vi "INI_Driver.vi"(0 "Data_In":string, 1 "Config_File_Path":path, 2 "Section":string, 5 "Key":string, 11 "Error_Out":errorcluster, 13 "INI_Operation_Select":T1=enum."Write") -> (4 "Data_Out":string, 6 "Key_Names":string[](array[string]), 15 "Error_Out":errorcluster)   [LabVIEW 2023]
doc: "Used to read and write the ini file"
uses:
  Controls/INI_Operation_Select.ctl
  <vilib>/Utility/config.llb/Read Key (String).vi
  <vilib>/Utility/config.llb/Write Key (String).vi
  <vilib>/Utility/config.llb/NI_LVConfig.lvlib
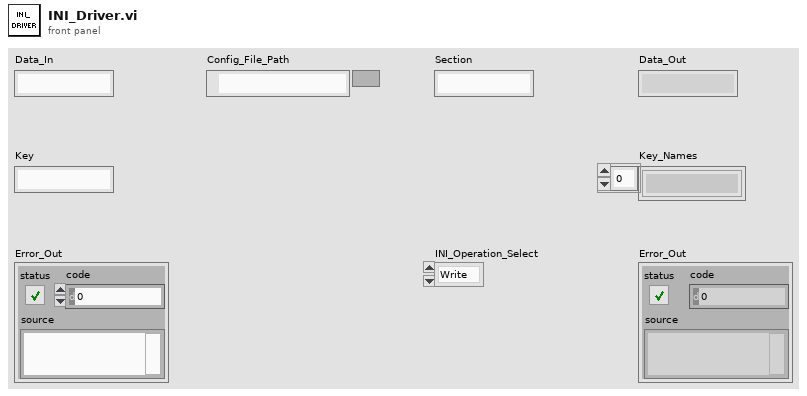
[diagram p1: front panel]
types:
  T1 = typedef "INI_Operation_Select.ctl" = enum16{"Initialize", "Read", "Read_Key", "Write"}
  T2 = typedef "NI_LVConfig.lvlib/Config Data RefNum.ctl" = refnum<k1>
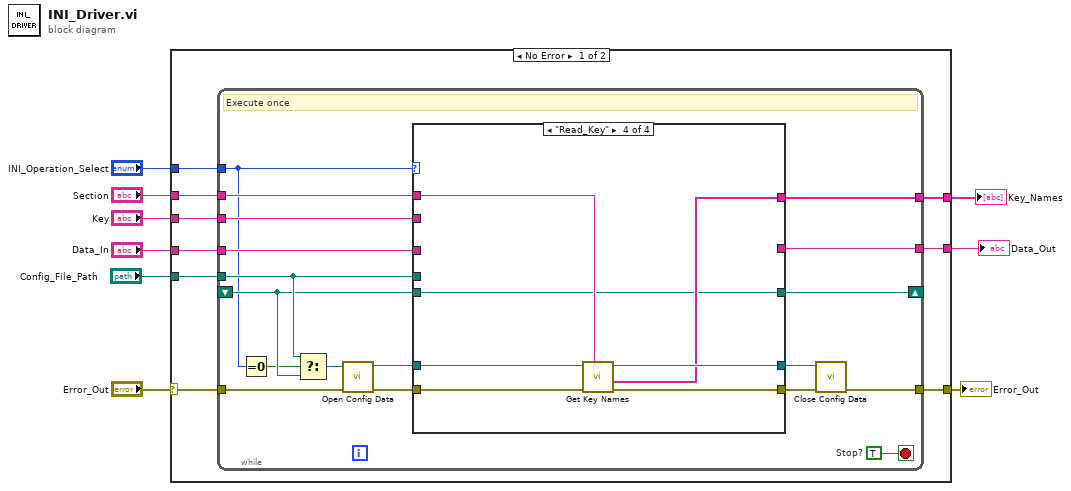
[diagram p0: block diagram]
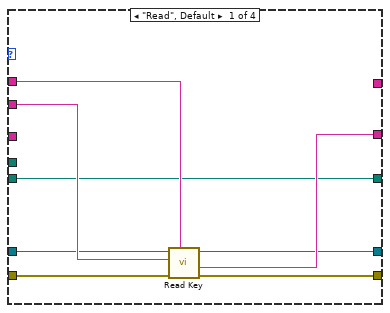
[diagram p2: hidden frame]
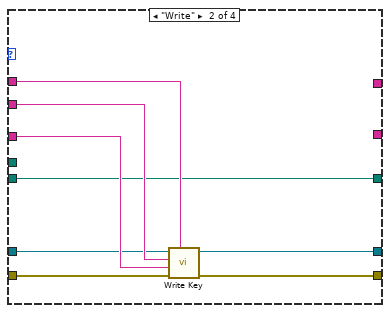
[diagram p3: hidden frame]
diagram:
  n1 = case shown="No Error" "Error_Out" {
    selector: "Error_Out" -> [w16 w63]
    tunnel: "INI_Operation_Select" -> [w18 _]
    tunnel: [w17 w63] -> w5
    tunnel: "Key" -> [w15 _]
    tunnel: "Section" -> [w14 _]
    tunnel: [w13 _] -> w4
    tunnel: "Data_In" -> [w12 _]
    tunnel: "Config_File_Path" -> [w10 _]
    tunnel: [w11 _] -> w1
    frame No Error {
      n2 = while {
        tunnel: w18 -> [w20]
        tunnel: [w26] -> w17
        tunnel: w16 -> [w30]
        tunnel: w15 -> [w36]
        tunnel: w14 -> [w35]
        tunnel: [w33] -> w13
        tunnel: w12 -> [w32]
        shift-right: [w25] -> _
        shift-left: _ -> [w21]
        tunnel: w10 -> [w22]
        tunnel: [w24] -> w11
        stop <- w34 stop-if-true
        w34 = TRUE  # Stop?
        # "Execute once"
        n3 = Equal To 0?(x=w20) -> (x = 0?=w19:bool)
        n4 = Select(t=w22, s=w19, f=w21) -> (s? t:f=w23:path)
        n5 = call <vilib>:"Open Config Data.vi"("error in (no error)"=w30, "configuration file path"=w23) -> ("error out"=w29:errorcluster, "refnum"=w31:T2)  [unwired: 7 in, 1 out]
        n6 = case shown="\"Read_Key\"" w20 {
          tunnel: [w38 w48 w55 w61] -> w27
          tunnel: w29 -> [w40 w49 w55 w62]
          tunnel: w36 -> [w44 w52 _ _]
          tunnel: w35 -> [w43 w51 _ w58]
          tunnel: [w42 _ _ _] -> w33
          tunnel: w32 -> [_ w50 _ _]
          tunnel: w22 -> [_ _ w54 _]
          tunnel: w31 -> [w41 w46 w53 w60]
          tunnel: [w39 w47 w53 w59] -> w28
          tunnel: [w37 w45 w54 w56] -> w25
          tunnel: w21 -> [w37 w45 _ w56]
          tunnel: [_ _ _ w57] -> w24
          frame "Read", Default {
            n7 = call-poly <vilib>:"Read Key.vi"("section"=w43, "error in (no error)"=w40, "key"=w44, "refnum"=w41) -> ("error out"=w38:errorcluster, "value"=w42:string, "refnum out"=w39:T2)  [unwired: 4 in, 1 out]
          }
          frame "Write" {
            n8 = call-poly <vilib>:"Write Key.vi"("section"=w51, "error in (no error)"=w49, "value"=w50, "key"=w52, "refnum"=w46) -> ("error out"=w48:errorcluster, "refnum out"=w47:T2)  [unwired: 4 in, 1 out]
          }
          frame "Initialize" {
          }
          frame "Read_Key" {
            n9 = call <vilib>:"Get Key Names.vi"("section"=w58, "error in (no error)"=w62, "refnum"=w60) -> ("error out"=w61:errorcluster, "key names"=w57:string[], "refnum out"=w59:T2)  [unwired: 5 in, 1 out]
          }
        }
        n10 = call <vilib>:"Close Config Data.vi"("error in (no error)"=w27, "refnum"=w28) -> ("error out"=w26:errorcluster)  [unwired: 8 in, 1 out]
      }
    }
    frame Error {
    }
  }
  "Error_Out" <- w5
  "Data_Out" <- w4
  "Key_Names" <- w1
